vi "ADCP_RREQ_Packet_To_Processed_Bytes.vi"(8 "error in (no error)":errorcluster, 10 "RREQ_Packet":T1, 11 "ADCP In":refnum<class "ADCP.lvclass">) -> (0 "error out":errorcluster, 2 "Processed Packet Bytes":u8[](array[numeric]), 3 "ADCP Out":refnum<class "ADCP.lvclass">)   [LabVIEW 2017, in "ADCP.lvclass"]
uses:
  ADCP.lvclass
  ADCP.lvclass/ADCP.ctl
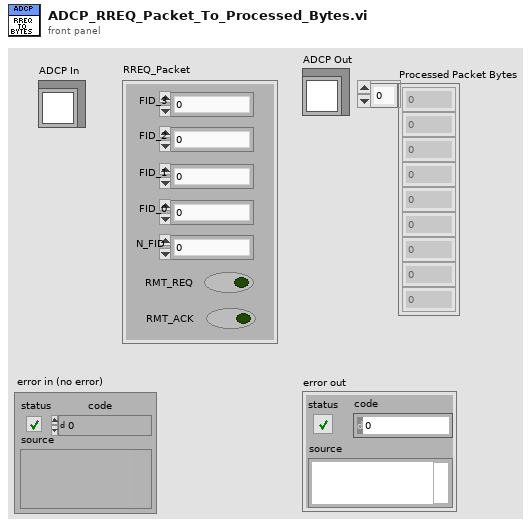
[diagram p1: front panel]
types:
  T1 = cluster{"FID_3":u8, "FID_2":u8, "FID_1":u8, "FID_0":u8, "N_FID":u8, "RMT_REQ":bool, "RMT_ACK":bool}
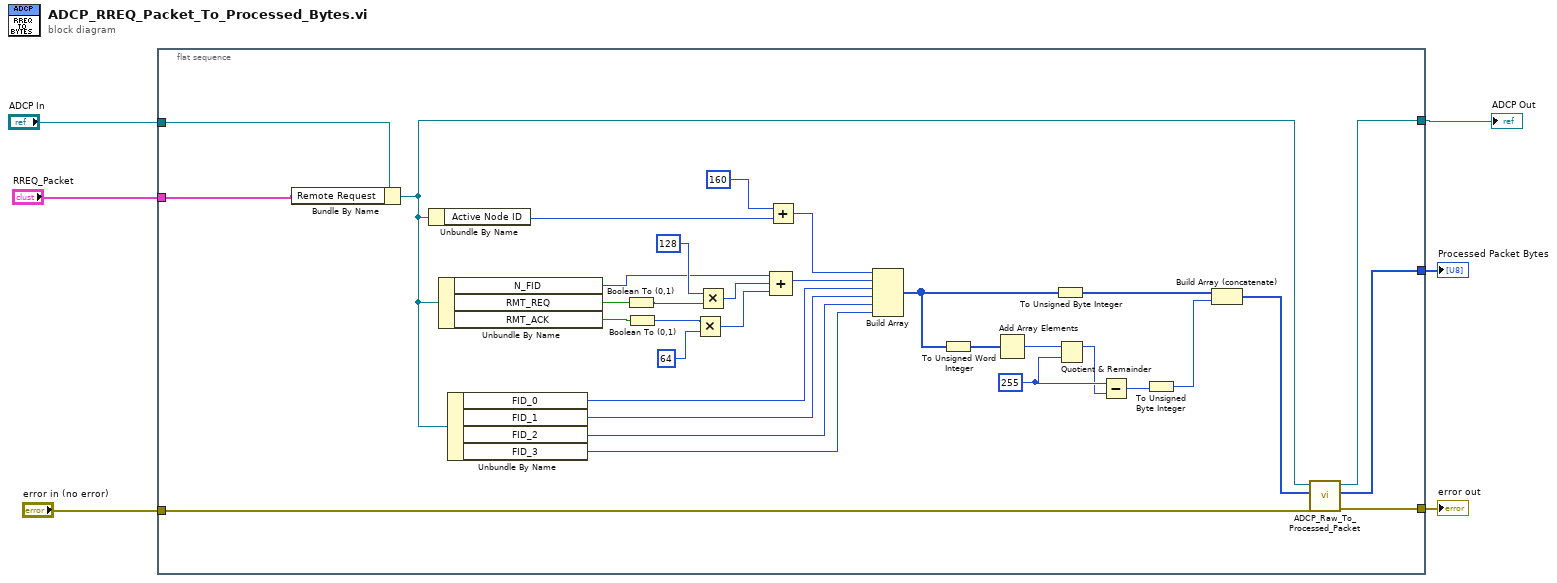
[diagram p0: block diagram]
diagram:
  n1 = flat-sequence {
    tunnel: "ADCP In" -> [w39]
    tunnel: "RREQ_Packet" -> [w38]
    tunnel: "error in (no error)" -> [w13]
    tunnel: [w11] -> w3
    tunnel: [w9] -> w1
    tunnel: [w8] -> w2
    frame #0 {
      w18 = u16 255 ("y")
      n2 = Bundle By Name(cluster=w39, "Remote Request"=w38) -> (w12:refnum<class "ADCP.lvclass">)
      n3 = Unbundle By Name(w12) -> ("Active Node ID"=w23:u8)
      n4 = Unbundle By Name(w12) -> ("N_FID"=w29:u8, "RMT_REQ"=w37:bool, "RMT_ACK"=w36:bool)
      n5 = Unbundle By Name(w12) -> ("FID_0"=w27:u8, "FID_1"=w26:u8, "FID_2"=w25:u8, "FID_3"=w24:u8)
      n6 = Boolean To (0,1)(Boolean=w37) -> (0, 1=w35:i16)
      n7 = Boolean To (0,1)(Boolean=w36) -> (0, 1=w33:i16)
      n8 = Multiply(x=w33, y=i16 64) -> (x*y=w30:i16)
      n9 = Multiply(x=i16 128, y=w35) -> (x*y=w31:i16)
      n10 = Add(x=u8 160, y=w23) -> (x+y=w22:u8)
      n11 = Compound Arithmetic op=ADD(w29, w31, w30) -> (w28:i16)
      n12 = Build Array(w22, w28, w27, w26, w25, w24) -> (w15:i16[])
      n13 = To Unsigned Word Integer(number=w15) -> (unsigned 16bit integer=w20:u16[])
      n14 = Add Array Elements(numeric array=w20) -> (sum=w19:u16)
      n15 = To Unsigned Byte Integer(number=w15) -> (unsigned 8bit integer=w7:u8[])
      n16 = Quotient & Remainder(x=w19, y=w18) -> (x-y*floor(x/y)=w17:u16)  [unwired: 1 out]
      n17 = Subtract(x=w18, y=w17) -> (x-y=w16:u16)
      n18 = To Unsigned Byte Integer(number=w16) -> (unsigned 8bit integer=w14:u8)
      n19 = Build Array (concatenate)(w7, w14) -> (w10:u8[])
      n20 = call "ADCP_Raw_To_Processed_Packet.vi"("error in (no error)"=w13, "Raw Packet"=w10, "ADCP in"=w12) -> ("error out"=w9:errorcluster, "Processed Packet"=w8:u8[], "ADCP out"=w11:refnum<class "ADCP.lvclass">)  [unwired: 6 in]
    }
  }
  "ADCP Out" <- w3
  "Processed Packet Bytes" <- w2
  "error out" <- w1
